vi "Configure Branch Counter Reset.vi"(8 "error in (no error)":errorcluster, 9 "Counter (0)":u32, 10 "Block Number (0)":u32, 11 "VISA resource name":refnum<visa-resource-name>) -> (0 "error out":errorcluster, 3 "VISA resource name out":refnum<visa-resource-name>)   [LabVIEW 2016, in "Keithley DMM6500 DAQ6500 Series.lvlib"]
doc: "Creates a block in the trigger model that resets a branch counter to 0. When the trigger model reaches the Counter Reset block, it resets the count of the specified Branch on Counter block to zero."
uses:
  Keithley DMM6500 DAQ6500 Series.lvlib
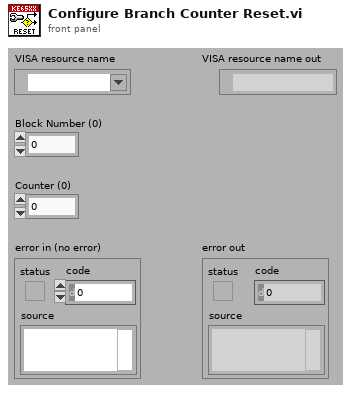
[diagram p1: front panel]
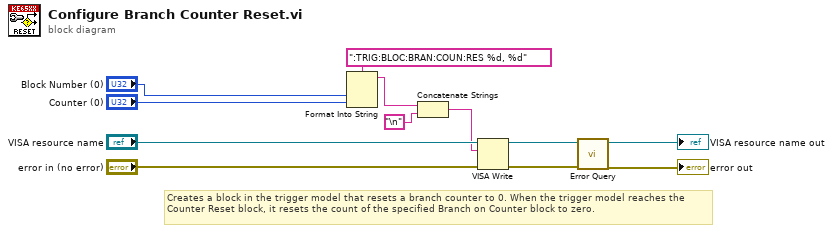
[diagram p0: block diagram]
diagram:
  # "Creates a block in the trigger model that resets a branch counter to 0. When the trigger model reaches the Counter Reset block, it resets the count of the specified Branch on Counter block to zero."
  n1 = Format Into String(format string=":TRIG:BLOC:BRAN:COUN:RES %d, %d", "Block Number (0)", "Counter (0)") -> (resulting string=w1:string)  [unwired: 2 in, 1 out]
  n2 = Concatenate Strings(w1, "\n") -> (w2:string)
  n3 = VISA Write(VISA resource name="VISA resource name", write buffer=w2, error in (no error)="error in (no error)") -> (VISA resource name out=w7:refnum<visa-resource-name>, error out=w6:errorcluster)  [unwired: 1 out]
  n4 = call "Error Query.vi"("error in (no error)"=w6, "VISA resource name"=w7) -> ("error out"=→"error out":errorcluster, "VISA resource name out"=→"VISA resource name out":refnum<visa-resource-name>)  [unwired: 6 in, 2 out]
